vi "RP100ToggleOutput.vi"(2 "error in (no error)":errorcluster, 3 "Enable?":bool, 4 "Source":enum16{"1", "2", "Both"}(ring), 5 "VISA resource name":refnum<visa-resource-name>) -> (0 "error out":errorcluster, 1 "VISA resource name out":refnum<visa-resource-name>)   [LabVIEW 2019, in "RP100.lvlib"]
uses:
  RP100.lvlib
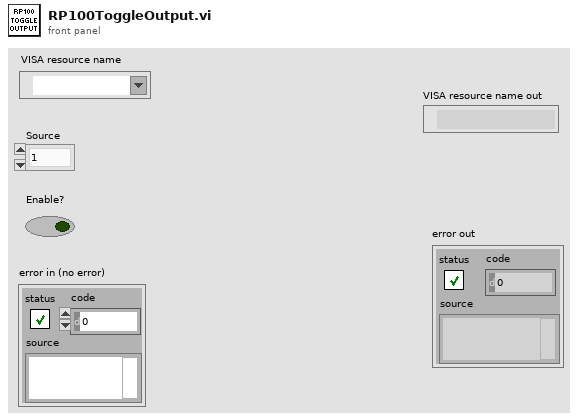
[diagram p1: front panel]
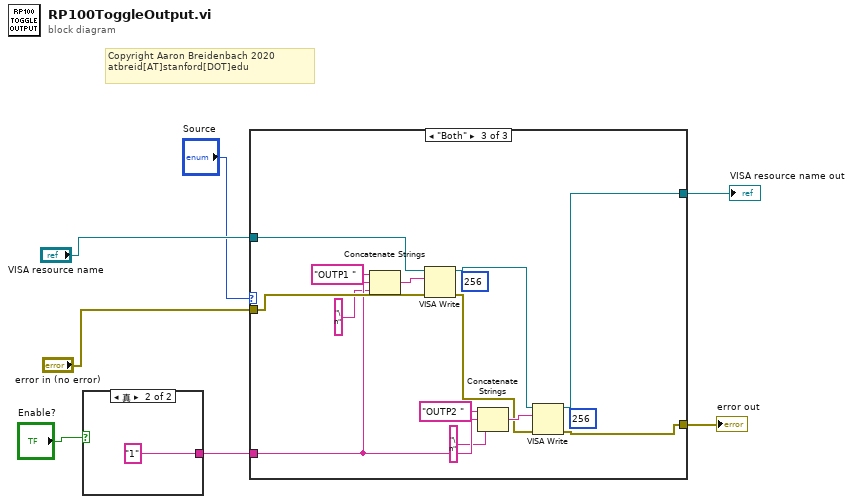
[diagram p0: block diagram]
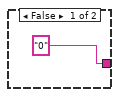
[diagram p2: hidden frame]
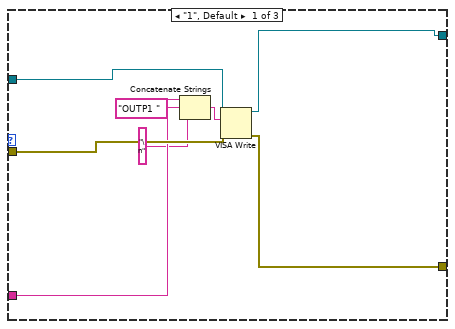
[diagram p3: hidden frame]
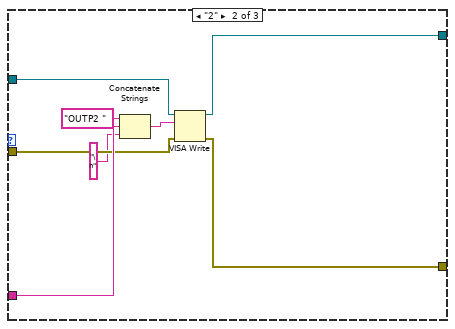
[diagram p4: hidden frame]
diagram:
  # "Copyright Aaron Breidenbach 2020\natbreid[AT]stanford[DOT]edu"
  n1 = case shown="真" "Enable?" {
    tunnel: ["0" "1"] -> w3
    frame False {
    }
    frame True {
    }
  }
  n2 = case shown="\"Both\"" "Source" {
    tunnel: w3 -> [w13 w24 w32]
    tunnel: "VISA resource name" -> [w15 w22 w35]
    tunnel: "error in (no error)" -> [w14 w21 w36]
    tunnel: [w10 w18 w27] -> w2
    tunnel: [w11 w19 w26] -> w1
    frame "1", Default {
      n3 = Concatenate Strings("OUTP1 " ("string"), w13, "\n" ("string")) -> (w17:string)
      n4 = VISA Write(VISA resource name=w15, write buffer=w17, error in (no error)=w14) -> (VISA resource name out=w11:refnum<visa-resource-name>, error out=w10:errorcluster)  [unwired: 1 out]
    }
    frame "2" {
      n5 = Concatenate Strings("OUTP2 " ("string"), w24, "\n" ("string")) -> (w25:string)
      n6 = VISA Write(VISA resource name=w22, write buffer=w25, error in (no error)=w21) -> (VISA resource name out=w19:refnum<visa-resource-name>, error out=w18:errorcluster)  [unwired: 1 out]
    }
    frame "Both" {
      (unwired) u32 256 ("byte count")
      (unwired) u32 256 ("byte count")
      n7 = Concatenate Strings("OUTP1 " ("string"), w32, "\n" ("string")) -> (w38:string)
      n8 = VISA Write(VISA resource name=w35, write buffer=w38, error in (no error)=w36) -> (VISA resource name out=w29:refnum<visa-resource-name>, error out=w28:errorcluster)  [unwired: 1 out]
      n9 = Concatenate Strings("OUTP2 " ("string"), w32, "\n" ("string")) -> (w34:string)
      n10 = VISA Write(VISA resource name=w29, write buffer=w34, error in (no error)=w28) -> (VISA resource name out=w26:refnum<visa-resource-name>, error out=w27:errorcluster)  [unwired: 1 out]
    }
  }
  "VISA resource name out" <- w1
  "error out" <- w2
